vi "Select TAG.vi"(8 "error in (no error)":errorcluster, 11 "input string":string) -> (0 "error out":errorcluster, 2 "number":i32, 3 "Tag":string)   [LabVIEW 2019]
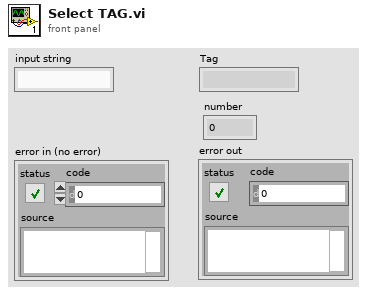
[diagram p1: front panel]
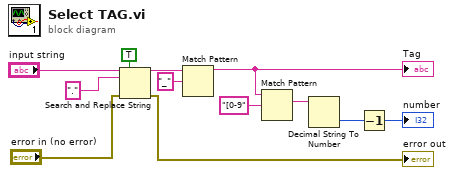
[diagram p0: block diagram]
diagram:
  n1 = Search and Replace String(replace all?=TRUE ("replace all? (F)"), input string="input string", search string=".", error in="error in (no error)") -> (result string=w9:string, error out=→"error out":errorcluster)  [unwired: 4 in, 2 out]
  n2 = Match Pattern(string=w9, regular expression="_") -> (before substring=w4:string)  [unwired: 1 in, 3 out]
  "Tag" <- w4
  n3 = Match Pattern(string=w4, regular expression="[0-9") -> (match substring=w3:string)  [unwired: 1 in, 3 out]
  n4 = Decimal String To Number(string=w3) -> (number=w2:i32)  [unwired: 2 in, 1 out]
  n5 = Decrement(x=w2) -> (x-1=→"number":i32)
